vi "TEST - Index 2D Array Elements.vi"(8 "error in (no error)":errorcluster) -> (0 "error out":errorcluster, 2 "Pass?":bool=TRUE)   [LabVIEW 2009]
doc: "This VI template can be used for the functional testing of VIs; this implementation includes handling for the testing of polymorphic VIs, and the polymorphic elements should be removed if not needed.\n\nCoded by Douglas A. Femec, January 24, 2006.\n\nCopyright (c) 2005-2006 MKS Instruments, Inc.\nAll rights reserved."
uses:
  TEST - Index 2D Array Elements - Inputs.ctl
  Polymorphizer+ Data Type.ctl
  TEST - Index 2D Array Elements - Outputs.ctl
  source/library/Index Array Elements/Index 2D Array Elements (EXT).vi
  source/library/Index Array Elements/Index 2D Array Elements (I64).vi
  source/library/Index Array Elements/Index 2D Array Elements (U64).vi
  source/library/Index Array Elements/Index 2D Array Elements (LVObject).vi
  source/library/Index Array Elements/Index 2D Array Elements (DBL).vi
  source/library/Index Array Elements/Index 2D Array Elements (SGL).vi
  source/library/Index Array Elements/Index 2D Array Elements (I32).vi
  source/library/Index Array Elements/Index 2D Array Elements (I16).vi
  source/library/Index Array Elements/Index 2D Array Elements (I8).vi
  source/library/Index Array Elements/Index 2D Array Elements (U32).vi
  source/library/Index Array Elements/Index 2D Array Elements (U16).vi
  source/library/Index Array Elements/Index 2D Array Elements (U8).vi
  source/library/Index Array Elements/Index 2D Array Elements (CXT).vi
  source/library/Index Array Elements/Index 2D Array Elements (CDB).vi
  source/library/Index Array Elements/Index 2D Array Elements (CSG).vi
  source/library/Index Array Elements/Index 2D Array Elements (Boolean).vi
  source/library/Index Array Elements/Index 2D Array Elements (String).vi
  source/library/Index Array Elements/Index 2D Array Elements (Path).vi
  source/library/Index Array Elements/Index 2D Array Elements (Variant).vi
  TestClass/TestClass.lvclass
panel:
  out "Generated Outputs":T1[][](array[typedef])=[[{"Description"="Expect empty array", "Elements"=[]}, {"Description"="Expect empty array", "Elements"=[]}, {"Description"="Expect empty array", "Elements"=[]}, {"Description"="Expect empty array", "Elements"=[]}, {"Description"="Expect empty array", "Elements"=[]}, {"Description"="Expect empty array", "Elements"=[]}, {"Description"="Expect empty array", "Elements"=[]}, {"Description"="Expect empty array", "Elements"=[]}, {"Description"="Expect empty array", "Elements"=[]}, {"Description"="Expect empty array", "Elements"=[]}, {"Description"="Expect empty array", "Elements"=[]}, {"Description"="Expect empty array", "Elements"=[]}, {"Description"="Expect empty array", "Elements"=[]}, {"Description"="Expect empty array", "Elements"=[]}, {"Description"="Expect empty array", "Elements"=[]}, {"Description"="Expect empty array", "Elements"=[]}], [{"Description"="Default data", "Elements"=[0.0, 0.0]}, {"Description"="Default data", "Elements"=[0.0, 0.0]}, {"Description"="Default data", "Elements"=[0.0, 0.0]}, {"Description"="Default data", "Elements"=[0.0, 0.0]}, {"Description"="Default data", "Elements"=[0.0, 0.0]}, {"Description"="Default data", "Elements"=[0.0, 0.0]}, {"Description"="Default data", "Elements"=[0.0, 0.0]}, {"Description"="Default data", "Elements"=[0.0, 0.0]}, {"Description"="Default data", "Elements"=[0.0, 0.0]}, {"Description"="Default data", "Elements"=[0.0, 0.0]}, {"Description"="Default data", "Elements"=[0.0, 0.0]}, {"Description"="Default data", "Elements"=[0.0, 0.0]}, {"Description"="Default data", "Elements"=[0.0, 0.0]}, {"Description"="Default data", "Elements"=[0.0, 0.0]}, {"Description"="Default data", "Elements"=[0.0, 0.0]}, {"Description"="Default data", "Elements"=[0.0, 0.0]}], [{"Description"="Expect some elements", "Elements"=[11.0]}, {"Description"="Expect some elements", "Elements"=[11.0]}, {"Description"="Expect some elements", "Elements"=[11.0]}, {"Description"="Expect some elements", "Elements"=[11.0]}, {"Description"="Expect some elements", "Elements"=[11.0]}, {"Description"="Expect some elements", "Elements"=[11.0]}, {"Description"="Expect some elements", "Elements"=[11.0]}, {"Description"="Expect some elements", "Elements"=[11.0]}, {"Description"="Expect some elements", "Elements"=[11.0]}, {"Description"="Expect some elements", "Elements"=[11.0]}, {"Description"="Expect some elements", "Elements"=[11.0]}, {"Description"="Expect some elements", "Elements"=[11.0]}, {"Description"="Expect some elements", "Elements"=[11.0]}, {"Description"="Expect some elements", "Elements"=[11.0]}, {"Description"="Expect some elements", "Elements"=[11.0]}, {"Description"="", "Elements"=[]}], [{"Description"=" diagonal, backwards", "Elements"=[8.0, 4.0, 0.0]}, {"Description"=" diagonal, backwards", "Elements"=[8.0, 4.0, 0.0]}, {"Description"=" diagonal, backwards", "Elements"=[8.0, 4.0, 0.0]}, {"Description"=" diagonal, backwards", "Elements"=[8.0, 4.0, 0.0]}, {"Description"=" diagonal, backwards", "Elements"=[8.0, 4.0, 0.0]}, {"Description"=" diagonal, backwards", "Elements"=[8.0, 4.0, 0.0]}, {"Description"=" diagonal, backwards", "Elements"=[8.0, 4.0, 0.0]}, {"Description"=" diagonal, backwards", "Elements"=[8.0, 4.0, 0.0]}, {"Description"=" diagonal, backwards", "Elements"=[8.0, 4.0, 0.0]}, {"Description"=" diagonal, backwards", "Elements"=[8.0, 4.0, 0.0]}, {"Description"=" diagonal, backwards", "Elements"=[8.0, 4.0, 0.0]}, {"Description"=" diagonal, backwards", "Elements"=[8.0, 4.0, 0.0]}, {"Description"=" diagonal, backwards", "Elements"=[8.0, 4.0, 0.0]}, {"Description"=" diagonal, backwards", "Elements"=[8.0, 4.0, 0.0]}, {"Description"=" diagonal, backwards", "Elements"=[8.0, 4.0, 0.0]}, {"Description"="", "Elements"=[]}]] {"Elements" format="%.2f"}
  in  "Expected Outputs":T1[](array[typedef])=[{"Description"="Expect empty array", "Elements"=[]}, {"Description"="Default data", "Elements"=[0.0, 0.0]}, {"Description"="Expect some elements", "Elements"=[11.0]}, {"Description"=" diagonal, backwards", "Elements"=[8.0, 4.0, 0.0]}] {"Elements" format="%.2f"}
  in  "Inputs":T2[](array[typedef])=[{"Description"="Empty indices array", "Data Types to Test"=[enum."EXT", enum."DBL", enum."SGL", enum."I32", enum."I16", enum."I8", enum."U32", enum."U16", enum."U8", enum."CXT", enum."CDB", enum."CSG", enum."Boolean", enum."String", enum."Path", enum."Variant", enum."I64", enum."U64", enum."LabVIEW Object"], "Array"=[[1.0, 2.0], [3.0, 4.0]], "Indices 0"=[], "Indices 1"=[]}, {"Description"="Empty input array", "Data Types to Test"=[enum."EXT", enum."DBL", enum."SGL", enum."I32", enum."I16", enum."I8", enum."U32", enum."U16", enum."U8", enum."CXT", enum."CDB", enum."CSG", enum."Boolean", enum."String", enum."Path", enum."Variant", enum."I64", enum."U64", enum."LabVIEW Object"], "Array"=[], "Indices 0"=[0, 1], "Indices 1"=[0, 1]}, {"Description"="", "Data Types to Test"=[enum."EXT", enum."DBL", enum."SGL", enum."I32", enum."I16", enum."I8", enum."U32", enum."U16", enum."U8", enum."CXT", enum."CDB", enum."CSG", enum."String", enum."Path", enum."Variant", enum."I64", enum."U64", enum."LabVIEW Object"], "Array"=[[1.0, 3.0], [5.0, 7.0], [9.0, 11.0]], "Indices 0"=[2], "Indices 1"=[1]}, {"Description"="Get diagonal, backwards", "Data Types to Test"=[enum."EXT", enum."DBL", enum."SGL", enum."I32", enum."I16", enum."I8", enum."U32", enum."U16", enum."U8", enum."CXT", enum."CDB", enum."CSG", enum."String", enum."Path", enum."Variant", enum."I64", enum."U64", enum."LabVIEW Object"], "Array"=[[0.0, 1.0, 2.0], [3.0, 4.0, 5.0], [6.0, 7.0, 8.0]], "Indices 0"=[2, 1, 0], "Indices 1"=[2, 1, 0]}] {"Array" format="%.2f"}
  # "Copyright (c) 2005-2006 MKS Instruments, Inc.\nAll rights reserved."
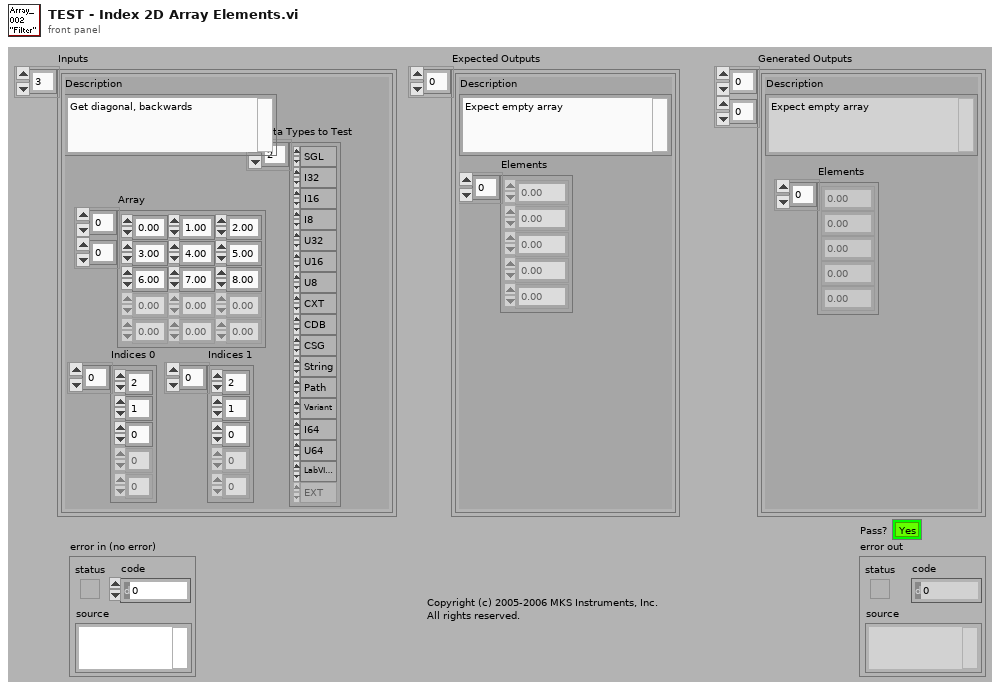
[diagram p1: front panel]
types:
  T1 = typedef "TEST - Index 2D Array Elements - Outputs.ctl" = cluster{"Description":string, "Elements":sgl[]}
  T2 = typedef "TEST - Index 2D Array Elements - Inputs.ctl" = cluster{"Description":string, "Data Types to Test":T3[], "Array":sgl[][], "Indices 0":i32[], "Indices 1":i32[]}
  T3 = typedef "Polymorphizer+ Data Type.ctl" = enum16{"EXT", "DBL", "SGL", "I32", "I16", "I8", "U32", "U16", "U8", "CXT", "CDB", "CSG", "Boolean", "String", "Path", "Variant", "CTL-REF", "GEN-REF", "GObj-REF", "VI-REF", "ENUM", "ERR", "FILE-REF", "MENU-REF", "MENU-RING", "PICT-RING", "TXT&PICT-RING", "TXT-RING", "I64", "U64", "LabVIEW Object"}
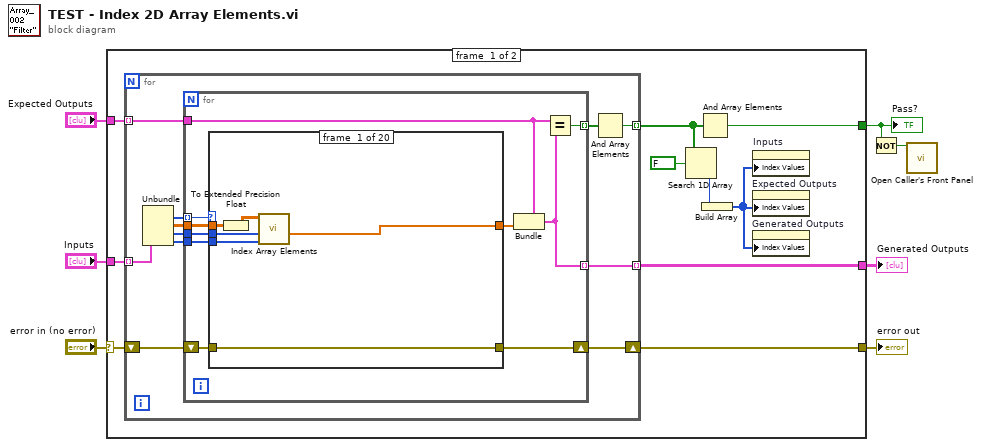
[diagram p0: block diagram]
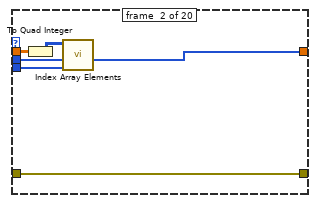
[diagram p2: hidden frame]
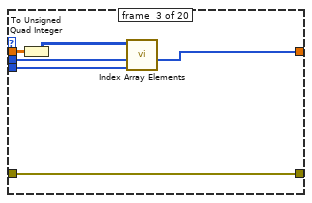
[diagram p3: hidden frame]
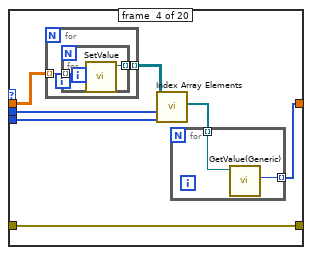
[diagram p4: hidden frame]
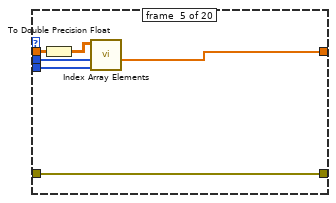
[diagram p5: hidden frame]
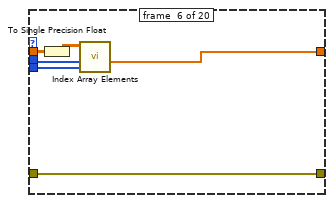
[diagram p6: hidden frame]
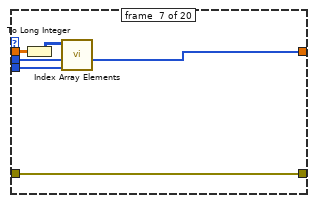
[diagram p7: hidden frame]
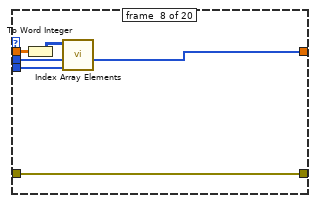
[diagram p8: hidden frame]
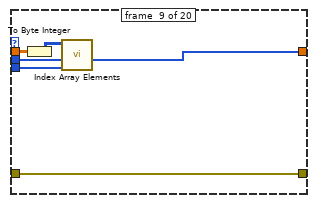
[diagram p9: hidden frame]
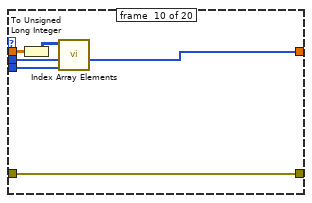
[diagram p10: hidden frame]
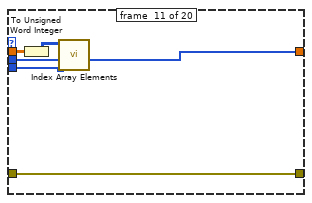
[diagram p11: hidden frame]
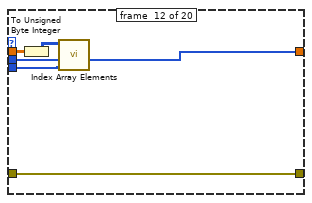
[diagram p12: hidden frame]
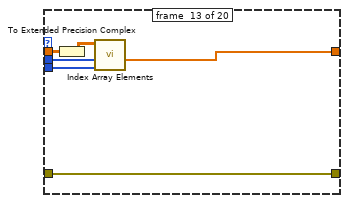
[diagram p13: hidden frame]
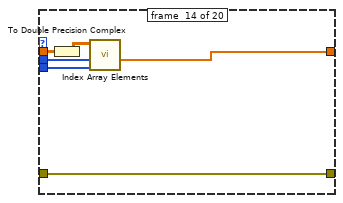
[diagram p14: hidden frame]
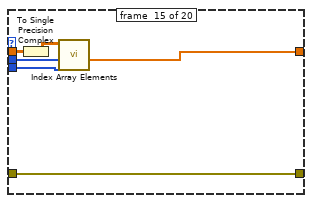
[diagram p15: hidden frame]
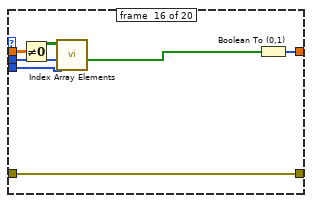
[diagram p16: hidden frame]
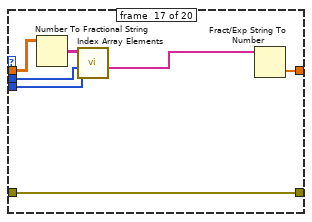
[diagram p17: hidden frame]
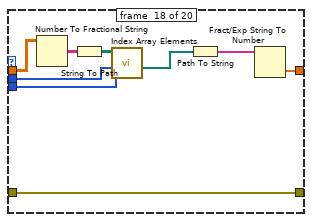
[diagram p18: hidden frame]
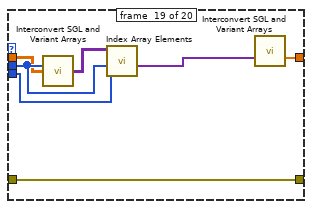
[diagram p19: hidden frame]
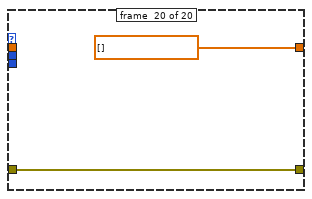
[diagram p20: hidden frame]
diagram:
  n1 = case shown="No Error" "error in (no error)" {
    selector: "error in (no error)" -> [w16 w168]
    tunnel: [w17 w168] -> w6
    tunnel: "Expected Outputs" -> [w14 _]
    tunnel: "Inputs" -> [w15 _]
    tunnel: [w13 _] -> w3
    tunnel: [w12 _] -> w2
    frame #0 {
      n2 = for {
        shift-right: [w23] -> w17
        shift-left: w16 -> [w24]
        tunnel: w15 -> [w25] mode=indexing
        tunnel: w14 -> [w28] mode=indexing
        tunnel: [w27] -> w13 mode=indexing
        tunnel: [w22] -> w11 mode=indexing
        n3 = Unbundle(w25) -> ("Data Types to Test"=w21:T3[], "Array"=w19:sgl[][], "Indices 0"=w20:i32[], "Indices 1"=w18:i32[])  [unwired: 1 out]
        n4 = for {
          tunnel: w28 -> [w38]
          tunnel: [w36] -> w27 mode=indexing
          tunnel: [w37] -> w26 mode=indexing
          shift-right: [w31] -> w23
          shift-left: w24 -> [w32]
          tunnel: w21 -> [w33] mode=indexing
          tunnel: w19 -> [w35]
          tunnel: w20 -> [w34]
          tunnel: w18 -> [w29]
          n5 = case shown="\"LabVIEW Object\"" w33 {
            tunnel: w35 -> [w44 w50 w56 w59 w75 w81 w87 w93 w99 w105 w111 w117 w123 w129 w135 w142 w149 w157 w161 _]
            tunnel: [w42 w48 w54 w57 w73 w79 w85 w91 w97 w103 w109 w115 w121 w127 w133 w141 w148 w156 w163 cxt[] []] -> w30
            tunnel: w34 -> [w40 w46 w52 w62 w72 w77 w84 w90 w96 w102 w108 w114 w120 w126 w132 w137 w145 w152 w162 _]
            tunnel: w32 -> [w43 w49 w55 w63 w74 w80 w86 w92 w98 w104 w110 w116 w122 w128 w134 w140 w147 w154 w165 w167]
            tunnel: [w43 w49 w55 w63 w74 w80 w86 w92 w98 w104 w110 w116 w122 w128 w134 w140 w147 w154 w165 w167] -> w31
            tunnel: w29 -> [w39 w45 w51 w61 w70 w76 w82 w88 w94 w100 w106 w112 w118 w124 w130 w136 w143 w150 w159 _]
            frame #0 {
              n6 = To Extended Precision Float(1:w44) -> (0:w41:ext[][])
              n7 = call-poly "Index Array Elements.vi"("indices 1"=w39, "indices 0"=w40, "array"=w41) -> ("elements"=w42:ext[])  [unwired: 8 in]
            }
            frame #1 {
              n8 = To Quad Integer(1:w50) -> (0:w47:i64[][])
              n9 = call-poly "Index Array Elements.vi"("indices 1"=w45, "indices 0"=w46, "array"=w47) -> ("elements"=w48:i64[])  [unwired: 8 in]
            }
            frame #2 {
              n10 = To Unsigned Quad Integer(1:w56) -> (0:w53:u64[][])
              n11 = call-poly "Index Array Elements.vi"("indices 1"=w51, "indices 0"=w52, "array"=w53) -> ("elements"=w54:u64[])  [unwired: 8 in]
            }
            frame #3 {
              n12 = for {
                tunnel: [w67] -> w60 mode=indexing
                tunnel: w59 -> [w66] mode=indexing
                n13 = for {
                  tunnel: [w69] -> w67 mode=indexing
                  tunnel: w66 -> [w68] mode=indexing
                  n14 = call "SetValue.vi"("Value"=w68) -> ("TestClass out"=w69:refnum<class "TestClass.lvclass">)  [unwired: 9 in, 1 out]
                }
              }
              n15 = call-poly "Index Array Elements.vi"("indices 1"=w61, "indices 0"=w62, "array"=w60) -> ("elements"=w58:refnum<class>[])  [unwired: 8 in]
              n16 = for {
                tunnel: w58 -> [w64] mode=indexing
                tunnel: [w65] -> w57 mode=indexing
                n17 = call "GetValue(Generic).vi"("TestClass in"=w64) -> ("Value"=w65:i32)  [unwired: 8 in, 2 out]
              }
            }
            frame #4 {
              n18 = To Double Precision Float(number=w75) -> (double precision float=w71:dbl[][])
              n19 = call-poly "Index Array Elements.vi"("indices 1"=w70, "indices 0"=w72, "array"=w71) -> ("elements"=w73:dbl[])  [unwired: 8 in]
            }
            frame #5 {
              n20 = To Single Precision Float(number=w81) -> (single precision float=w78:sgl[][])
              n21 = call-poly "Index Array Elements.vi"("indices 1"=w76, "indices 0"=w77, "array"=w78) -> ("elements"=w79:sgl[])  [unwired: 8 in]
            }
            frame #6 {
              n22 = To Long Integer(number=w87) -> (32bit integer=w83:i32[][])
              n23 = call-poly "Index Array Elements.vi"("indices 1"=w82, "indices 0"=w84, "array"=w83) -> ("elements"=w85:i32[])  [unwired: 8 in]
            }
            frame #7 {
              n24 = To Word Integer(number=w93) -> (16bit integer=w89:i16[][])
              n25 = call-poly "Index Array Elements.vi"("indices 1"=w88, "indices 0"=w90, "array"=w89) -> ("elements"=w91:i16[])  [unwired: 8 in]
            }
            frame #8 {
              n26 = To Byte Integer(number=w99) -> (8bit integer=w95:i8[][])
              n27 = call-poly "Index Array Elements.vi"("indices 1"=w94, "indices 0"=w96, "array"=w95) -> ("elements"=w97:i8[])  [unwired: 8 in]
            }
            frame #9 {
              n28 = To Unsigned Long Integer(number=w105) -> (unsigned 32bit integer=w101:u32[][])
              n29 = call-poly "Index Array Elements.vi"("indices 1"=w100, "indices 0"=w102, "array"=w101) -> ("elements"=w103:u32[])  [unwired: 8 in]
            }
            frame #10 {
              n30 = To Unsigned Word Integer(number=w111) -> (unsigned 16bit integer=w107:u16[][])
              n31 = call-poly "Index Array Elements.vi"("indices 1"=w106, "indices 0"=w108, "array"=w107) -> ("elements"=w109:u16[])  [unwired: 8 in]
            }
            frame #11 {
              n32 = To Unsigned Byte Integer(number=w117) -> (unsigned 8bit integer=w113:u8[][])
              n33 = call-poly "Index Array Elements.vi"("indices 1"=w112, "indices 0"=w114, "array"=w113) -> ("elements"=w115:u8[])  [unwired: 8 in]
            }
            frame #12 {
              n34 = To Extended Precision Complex(1:w123) -> (0:w119:cxt[][])
              n35 = call-poly "Index Array Elements.vi"("indices 1"=w118, "indices 0"=w120, "array"=w119) -> ("elements"=w121:cxt[])  [unwired: 8 in]
            }
            frame #13 {
              n36 = To Double Precision Complex(1:w129) -> (0:w125:cdb[][])
              n37 = call-poly "Index Array Elements.vi"("indices 1"=w124, "indices 0"=w126, "array"=w125) -> ("elements"=w127:cdb[])  [unwired: 8 in]
            }
            frame #14 {
              n38 = To Single Precision Complex(1:w135) -> (0:w131:csg[][])
              n39 = call-poly "Index Array Elements.vi"("indices 1"=w130, "indices 0"=w132, "array"=w131) -> ("elements"=w133:csg[])  [unwired: 8 in]
            }
            frame #15 {
              n40 = Not Equal To 0?(x=w142) -> (x != 0?=w138:bool[][])
              n41 = call-poly "Index Array Elements.vi"("indices 1"=w136, "indices 0"=w137, "array"=w138) -> ("elements"=w139:bool[])  [unwired: 8 in]
              n42 = Boolean To (0,1)(Boolean=w139) -> (0, 1=w141:i16[])
            }
            frame #16 {
              n43 = Number To Fractional String(number=w149) -> (F-format string=w144:string[][])  [unwired: 3 in]
              n44 = call-poly "Index Array Elements.vi"("indices 1"=w143, "indices 0"=w145, "array"=w144) -> ("elements"=w146:string[])  [unwired: 8 in]
              n45 = Fract/Exp String To Number(string=w146) -> (number=w148:dbl[])  [unwired: 3 in, 1 out]
            }
            frame #17 {
              n46 = Number To Fractional String(number=w157) -> (F-format string=w158:string[][])  [unwired: 3 in]
              n47 = String To Path(string=w158) -> (path=w151:path[][])
              n48 = call-poly "Index Array Elements.vi"("indices 1"=w150, "indices 0"=w152, "array"=w151) -> ("elements"=w153:path[])  [unwired: 8 in]
              n49 = Path To String(path=w153) -> (string=w155:string[])
              n50 = Fract/Exp String To Number(string=w155) -> (number=w156:dbl[])  [unwired: 3 in, 1 out]
            }
            frame #18 {
              n51 = call "Interconvert SGL and Variant Arrays.vi"("SGL 1D Array 2 In"=w162, "SGL 2D Array In"=w161) -> ("Variant 2D Array Out"=w160:variant[][])  [unwired: 9 in, 4 out]
              n52 = call-poly "Index Array Elements.vi"("indices 1"=w159, "indices 0"=w162, "array"=w160) -> ("elements"=w164:variant[])  [unwired: 8 in]
              n53 = call "Interconvert SGL and Variant Arrays.vi"("Variant 1D Array In"=w164) -> ("SGL 1D Array Out"=w163:sgl[])  [unwired: 10 in, 4 out]
            }
            frame #19 {
            }
          }
          n54 = Bundle(cluster=w38, "Elements"=w30) -> (w36:T1)  [unwired: 1 in]
          n55 = Equal?(x=w38, y=w36) -> (x = y?=w37:bool)
        }
        n56 = And Array Elements(Boolean array=w26) -> (logical AND=w22:bool)
      }
      n57 = Search 1D Array(1D array=w11, element=FALSE) -> (index of element=w9:i32)  [unwired: 1 in]
      n58 = And Array Elements(Boolean array=w11) -> (logical AND=w12:bool)
      n59 = Build Array(w9) -> (w8:i32[])
      n60 = property on="Inputs" class="Arr (strict)"("Index Values"=w8) -> ()  [unwired: 2 in, 2 out]
      n61 = property on="Expected Outputs" class="Arr (strict)"("Index Values"=w8) -> ()  [unwired: 2 in, 2 out]
      n62 = property on="Generated Outputs" class="Arr (strict)"("Index Values"=w8) -> ()  [unwired: 2 in, 2 out]
    }
    frame #1 {
    }
  }
  "error out" <- w6
  "Pass?" <- w2
  "Generated Outputs" <- w3
  n63 = Not(x=w2) -> (.not. x?=w1:bool)
  n64 = call "Open Caller's Front Panel.vi"("Open?"=w1) -> ()  [unwired: 14 in, 1 out]
